vi "Teleop.vi"(10 "Match Info":T1={"Autonomous Elapsed Seconds"=0.0, "TeleOp Elapsed Seconds"=0.0, "Disabled Elapsed Seconds"=0.0, "Visited Autonomous"=FALSE, "Visited TeleOp"=FALSE, "Visited Disabled"=FALSE, "Autonomous Settings"={"Autonomous Style"=enum."Independent", "VI Refnum"=refnum}}, 11 "Call Context":T2) -> ()   [LabVIEW 2017]
doc: "This VI is called for each TeleOp packet received from the DS where the robot is not disabled. It is often used to read from the joysticks and update I/O or to update setpoints for timed control loops. It should complete and return within 20 milliseconds or it may miss DS packets."
uses:
  <vilib>/Rock Robotics/WPI/DriverStation/WPI_DriverStationDerivedRobotMode.ctl
  <vilib>/Rock Robotics/WPI/DriverStation/WPI_DriverStationMatch Info.ctl
  <vilib>/Rock Robotics/Network Tables/NT Read Boolean.vi
  <vilib>/Rock Robotics/Network Tables/NT Read Number.vi
  <vilib>/Rock Robotics/WPI/Utilities/WPI_GetSetVariantRefNum.vi
  <vilib>/Rock Robotics/WPI/Solenoid/Deprecated/WPI_SolenoidSetBool.vi
  <vilib>/Rock Robotics/Network Tables/NT Write Numeric Array.vi
  <vilib>/Rock Robotics/Network Tables/NT Write Boolean Array.vi
panel:
  out "right direction":bool
  out "right distance":dbl
  out "left direction":bool
  out "left distance":dbl
  out "Sample Slider 0":dbl(slide) scale=0.0..5.0
  out "Sample Boolean 1":bool
  out "Sample Boolean 0":bool
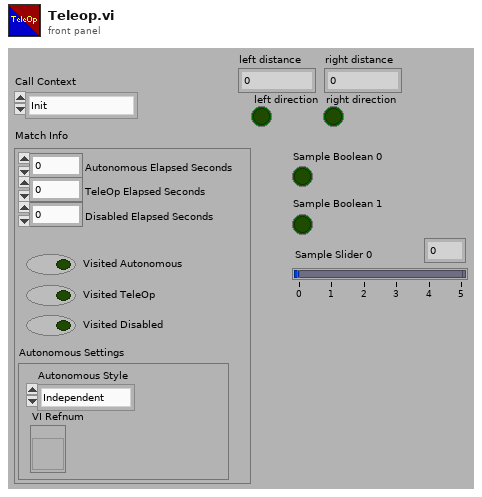
[diagram p1: front panel]
types:
  T1 = typedef "WPI_DriverStationMatch Info.ctl" = cluster{"Autonomous Elapsed Seconds":dbl, "TeleOp Elapsed Seconds":dbl, "Disabled Elapsed Seconds":dbl, "Visited Autonomous":bool, "Visited TeleOp":bool, "Visited Disabled":bool, "Autonomous Settings":cluster{"Autonomous Style":enum16{"Iterative", "Independent"}, "VI Refnum":refnum<vi>}}
  T2 = typedef "WPI_DriverStationDerivedRobotMode.ctl" = enum16{"Init", "Execute", "Stop"}
  T3 = typedef "WPI_EncoderDevRef.ctl" = cluster{"DevStatus":errorcluster, "EncoderIndex":T4, "CounterIndex":T5, "DistancePerCount":dbl, "Decoding Type":T6}
  T4 = typedef "FPGA_EncoderIdx.ctl" = enum8{"Enc 0", "Enc 1", "Enc 2", "Enc 3", "Enc 4", "Enc 5", "Enc 6", "Enc 7", "Invalid"}
  T5 = typedef "FPGA_CounterCtrSystemIndex.ctl" = enum8{"Ctr 0", "Ctr 1", "Ctr 2", "Ctr 3", "Ctr 4", "Ctr 5", "Ctr 6", "Ctr 7", "Invalid"}
  T6 = typedef "WPI_EncoderType.ctl" = enum16{"1x", "2x", "4x"}
  T7 = typedef "WPI_JoystickDevRef.ctl" = cluster{"Device":T8}
  T8 = typedef "WPI_JoystickDeviceEnum.ctl" = enum16{"USB 0", "USB 1", "USB 2", "USB 3", "USB 4", "USB 5"}
  T9 = typedef "WPI_RobotDriveDevRef.ctl" = cluster{"DevStatus":errorcluster, "Motors[]":T10[], "Square Inputs":bool, "Max Output":dbl}
  T10 = typedef "WPI_MotorControlDeviceRef.ctl" = cluster{"DeviceStatus":errorcluster, "Type":T11, "PWM":cluster{"PWM Channel":T12, "DeadBand":T13}, "CAN":cluster{"Device Number":u8, "SetOutput VI Ref":variant, "GetOutput VI Ref":variant, "Enable VI Ref":variant, "Disable VI Ref":variant, "Data":variant}, "Invert":bool, "DIO PWM":cluster{"PWM \"Enable\" Channel":T12, "DIOChannel":T14, "PWM Rate":dbl}}
  T11 = typedef "WPI_MotorControlType.ctl" = enum16{"PWM", "CAN", "DIO PWM"}
  T12 = typedef "FPGA_DIOPWMChannel.ctl" = enum8{"PWM 0", "PWM 1", "PWM 2", "PWM 3", "PWM 4", "PWM 5", "PWM 6", "PWM 7", "PWM 8", "PWM 9", "PWM MXP 0", "PWM MXP 1", "PWM MXP 2", "PWM MXP 3", "PWM MXP 4", "PWM MXP 5", "PWM MXP 6", "PWM MXP 7", "PWM MXP 8", "PWM MXP 9", "Invalid"}
  T13 = typedef "WPI_PWMDeadband.ctl" = cluster{"Name":string, "maxPositivePwm":i32, "minPositivePwm":i32, "centerPwm":i32, "maxNegativePwm":i32, "minNegativePwm":i32, "angularRange":u16}
  T14 = typedef "FPGA_DIOChannel.ctl" = enum8{"DIO 0", "DIO 1", "DIO 2", "DIO 3", "DIO 4", "DIO 5", "DIO 6", "DIO 7", "DIO 8", "DIO 9", "DIO MXP 0", "DIO MXP 1", "DIO MXP 2", "DIO MXP 3", "DIO MXP 4", "DIO MXP 5", "DIO MXP 6", "DIO MXP 7", "DIO MXP 8", "DIO MXP 9", "DIO MXP 10", "DIO MXP 11", "DIO MXP 12", "DIO MXP 13", "DIO MXP 14", "DIO MXP 15", "SPI Port CS1", "SPI Port CS2", "SPI Port CS3", "SPI Port MISO", "SPI Port MOSI", "Invalid"}
  T15 = cluster{"Buttons[0]":bool, "Buttons[1]":bool, "Buttons[2]":bool, "Buttons[3]":bool, "Buttons[4]":bool, "Buttons[5]":bool, "Buttons[6]":bool, "Buttons[7]":bool, "Buttons[8]":bool}
  T16 = typedef "WPI_SolenoidDevRef.ctl" = cluster{"DevStatus":errorcluster, "Pneumatics Control Module":u8, "Forward Solenoid Channel":T17, "Reverse Solenoid Channel":T17}
  T17 = typedef "WPI_SolenoidChannel.ctl" = enum8{"Solenoid 0", "Solenoid 1", "Solenoid 2", "Solenoid 3", "Solenoid 4", "Solenoid 5", "Solenoid 6", "Solenoid 7", "Invalid"}
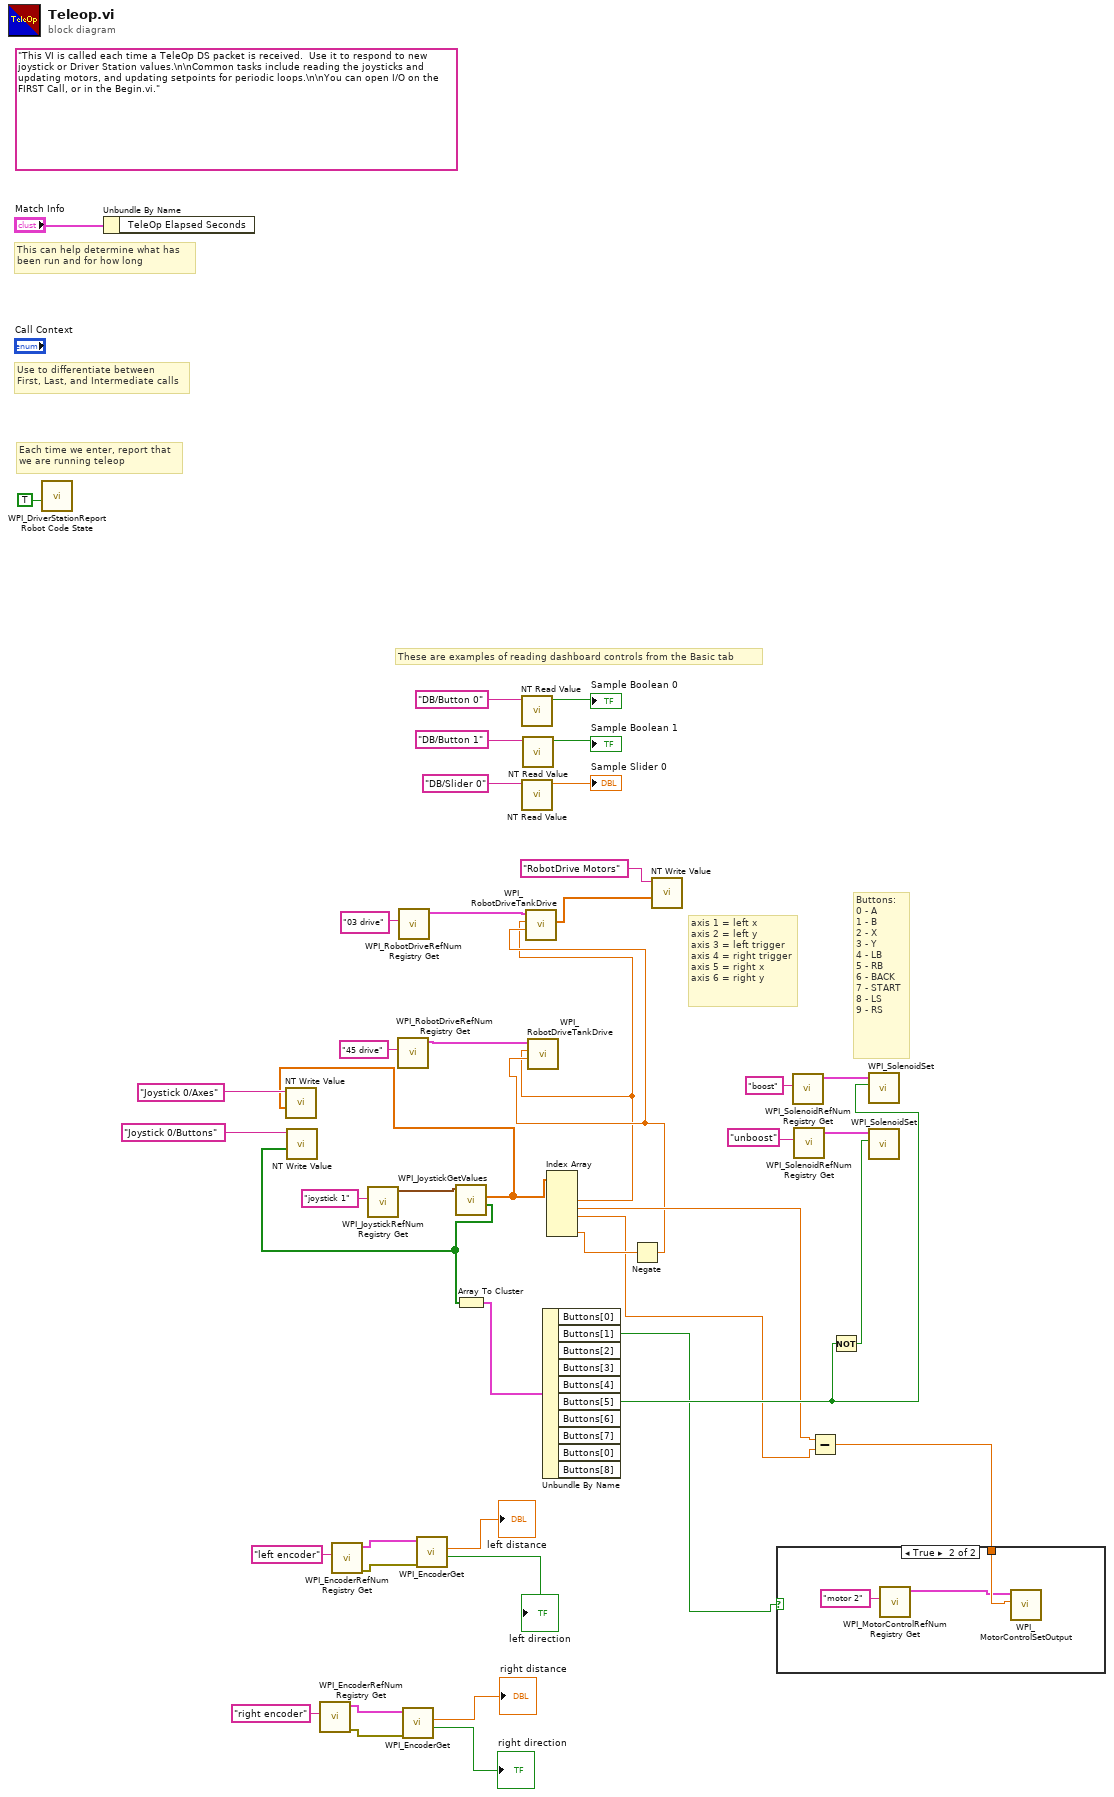
[diagram p0: block diagram]
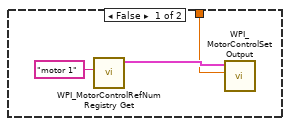
[diagram p2: hidden frame]
diagram:
  (unwired) "This VI is called each time a TeleOp DS packet is received.  Use it to respond to new joystick or Driver Station values.\n\nCommon tasks include reading the joysticks and updating motors, and updating setpoints for periodic loops.\n\nYou can open I/O on the FIRST Call, or in the Begin.vi."
  # "axis 1 = left x\naxis 2 = left y\naxis 3 = left trigger \naxis 4 = right trigger\naxis 5 = right x\naxis 6 = right y"
  # "Buttons:\n0 - A\n1 - B\n2 - X\n3 - Y\n4 - LB\n5 - RB\n6 - BACK\n7 - START\n8 - LS\n9 - RS"
  # "These are examples of reading dashboard controls from the Basic tab"
  # "Each time we enter, report that\nwe are running teleop"
  # "Use to differentiate between\nFirst, Last, and Intermediate calls"
  # "This can help determine what has\nbeen run and for how long"
  n1 = call <vilib>:"WPI_DriverStationReport Robot Code State.vi"("TeleOp"=TRUE ("Autonomous")) -> ()  [unwired: 10 in, 1 out]
  n2 = Unbundle By Name("Match Info") -> ()  [unwired: 1 out]
  n3 = call <vilib>:"WPI_EncoderRefNum Registry Get.vi"("refnum name"="right encoder") -> ("error out"=w9:errorcluster, "EncoderDevRef"=w12:T3)  [unwired: 9 in]
  n4 = call <vilib>:"WPI_EncoderRefNum Registry Get.vi"("refnum name"="left encoder") -> ("error out"=w10:errorcluster, "EncoderDevRef"=w11:T3)  [unwired: 9 in]
  n5 = call <vilib>:"WPI_JoystickRefNum Registry Get.vi"("refnum name"="joystick 1") -> ("JoystickDevRef"=w24:T7)  [unwired: 9 in, 1 out]
  n6 = call <vilib>:"WPI_RobotDriveRefNum Registry Get.vi"("refnum name"="45 drive") -> ("RobotDriveDevRef"=w22:T9)  [unwired: 9 in, 1 out]
  n7 = call <vilib>:"WPI_RobotDriveRefNum Registry Get.vi"("refnum name"="03 drive") -> ("RobotDriveDevRef"=w20:T9)  [unwired: 9 in, 1 out]
  n8 = call <vilib>:"WPI_EncoderGet.vi"("error in (no error)"=w9, "EncoderDevRef"=w12) -> ("Direction"=→"right direction":bool, "Distance"=→"right distance":dbl)  [unwired: 4 in, 4 out]
  n9 = call <vilib>:"WPI_EncoderGet.vi"("error in (no error)"=w10, "EncoderDevRef"=w11) -> ("Direction"=→"left direction":bool, "Distance"=→"left distance":dbl)  [unwired: 4 in, 4 out]
  n10 = call <vilib>:"WPI_JoystickGetValues.vi"("JoystickDevRef"=w24) -> ("Buttons"=w14:bool[], "Axes"=w13:dbl[])  [unwired: 6 in, 3 out]
  n11 = call-poly <vilib>:"NT Write Value.vi"("Numeric Array"=w13, "Name"="Joystick 0/Axes") -> ()  [unwired: 9 in, 1 out]
  n12 = call-poly <vilib>:"NT Write Value.vi"("Boolean Array"=w14, "Name"="Joystick 0/Buttons") -> ()  [unwired: 9 in, 1 out]
  n13 = Array To Cluster(array=w14) -> (cluster=w28:T15)
  n14 = call-poly <vilib>:"NT Read Value.vi"("Name"="DB/Button 0" ("refnum name")) -> ("Boolean"=→"Sample Boolean 0":bool)  [unwired: 9 in, 1 out]
  n15 = call-poly <vilib>:"NT Read Value.vi"("Name"="DB/Slider 0" ("refnum name")) -> ("Numeric"=→"Sample Slider 0":dbl)  [unwired: 9 in, 1 out]
  n16 = call-poly <vilib>:"NT Read Value.vi"("Name"="DB/Button 1" ("refnum name")) -> ("Boolean"=→"Sample Boolean 1":bool)  [unwired: 9 in, 1 out]
  n17 = Unbundle By Name(w28) -> ("Buttons[1]"=w2:bool, "Buttons[5]"=w36:bool)  [unwired: 8 out]
  n18 = Index Array(array=w13) -> (element #2=w25:dbl, element #3=w34:dbl, element #4=w1:dbl, element #6=w26:dbl)  [unwired: 6 in, 2 out]
  n19 = Negate(x=w26) -> (-x=w27:dbl)
  n20 = call <vilib>:"WPI_RobotDriveTankDrive.vi"("Right axis value"=w27, "Left axis value"=w25, "RobotDriveDevRef"=w20) -> ("Motor Values"=w17:dbl[])  [unwired: 6 in, 2 out]
  n21 = call <vilib>:"WPI_RobotDriveTankDrive.vi"("Right axis value"=w27, "Left axis value"=w25, "RobotDriveDevRef"=w22) -> ()  [unwired: 6 in, 3 out]
  n22 = call-poly <vilib>:"NT Write Value.vi"("Numeric Array"=w17, "Name"="RobotDrive Motors") -> ()  [unwired: 9 in, 1 out]
  n23 = call <vilib>:"WPI_SolenoidRefNum Registry Get.vi"("refnum name"="boost") -> ("SolenoidDevRef"=w31:T16)  [unwired: 9 in, 1 out]
  n24 = call <vilib>:"WPI_SolenoidRefNum Registry Get.vi"("refnum name"="unboost") -> ("SolenoidDevRef"=w32:T16)  [unwired: 9 in, 1 out]
  n25 = Subtract(x=w34, y=w1) -> (x-y=w35:dbl)
  n26 = case shown="True" w2 {
    tunnel: w35 -> [w45 w50]
    frame False {
      n27 = call <vilib>:"WPI_MotorControlRefNum Registry Get.vi"("refnum name"="motor 1") -> ("MotorControlDevRef"=w47:T10)  [unwired: 9 in, 1 out]
      n28 = call <vilib>:"WPI_MotorControlSetOutput.vi"("Output"=w45, "MotorControlDevRef"=w47) -> ()  [unwired: 7 in, 3 out]
    }
    frame True {
      n29 = call <vilib>:"WPI_MotorControlRefNum Registry Get.vi"("refnum name"="motor 2") -> ("MotorControlDevRef"=w49:T10)  [unwired: 9 in, 1 out]
      n30 = call <vilib>:"WPI_MotorControlSetOutput.vi"("Output"=w50, "MotorControlDevRef"=w49) -> ()  [unwired: 7 in, 3 out]
    }
  }
  n31 = Not(x=w36) -> (.not. x?=w33:bool)
  n32 = call-poly <vilib>:"WPI_SolenoidSet.vi"("Value"=w36, "SolenoidDevRef"=w31) -> ()  [unwired: 8 in, 2 out]
  n33 = call-poly <vilib>:"WPI_SolenoidSet.vi"("Value"=w33, "SolenoidDevRef"=w32) -> ()  [unwired: 8 in, 2 out]
